vi "test sv.vi"() -> ()   [LabVIEW 2018]
panel:
  out "Indices out":i32[](array[numeric])
  out "Data out":dbl[](array[numeric])
  in  "Data":dbl[](array[numeric])
  in  "Indices":i32[](array[numeric])
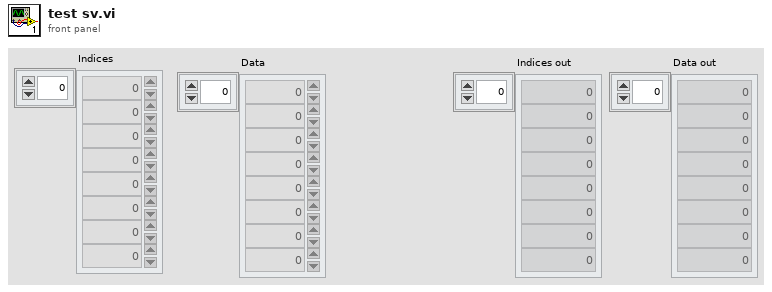
[diagram p1: front panel]
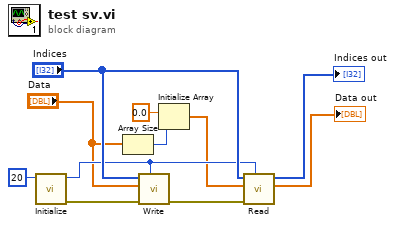
[diagram p0: block diagram]
diagram:
  n1 = call "Initialize.vi"("Size"=20) -> ("Error Out"=w10:errorcluster, "Map id"=w7:i32)  [unwired: 9 in]
  n2 = Array Size(array="Data") -> (size(s)=w4:i32)
  n3 = call "Write.vi"("Map id"=w7, "Error In"=w10, "Data"="Data", "Indices"="Indices") -> ("Error Out"=w9:errorcluster)  [unwired: 7 in]
  n4 = Initialize Array(0.0 ("element"), w4) -> (w3:dbl[])
  n5 = call "Read.vi"("Map id"=w7, "Error In"=w9, "Data in"=w3, "Indices in"="Indices") -> ("Data out"=→"Data out":dbl[], "Indices out"=→"Indices out":i32[])  [unwired: 5 in, 1 out]
